vi "Get Service.vi"(7 "Service Type":refnum<class "Service.lvclass">, 8 "error in (no error)":errorcluster, 11 "Values in":refnum<class "Values.lvclass">) -> (0 "error out":errorcluster, 2 "Service":refnum<class "Service.lvclass">, 3 "Values out":refnum<class "Values.lvclass">)   [LabVIEW 2020, in "HTTP Server.lvlib" / "Values.lvclass"]
uses:
  Values.lvclass
  Values.lvclass/Values.ctl
  Service/Service.lvclass
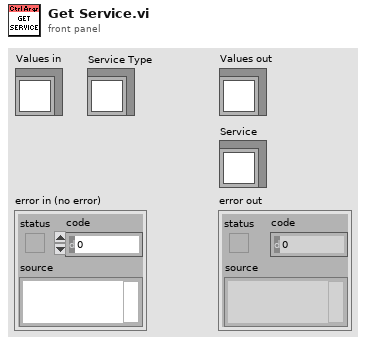
[diagram p1: front panel]
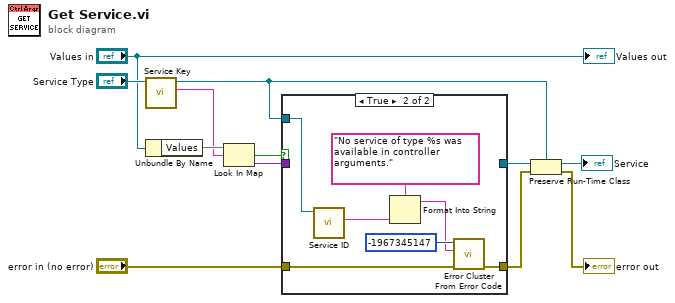
[diagram p0: block diagram]
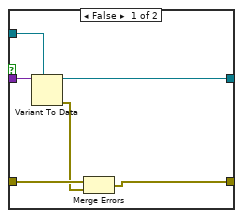
[diagram p2: hidden frame]
diagram:
  n1 = call "Service Key.vi"("Service In"="Service Type") -> ("Service Key"=w9:string, "Service"=w4:refnum<class "Service.lvclass">)  [unwired: 9 in]
  n2 = Unbundle By Name("Values in") -> ("Values"=w10:map{string, variant})
  n3 = Look In Map(map=w10, key=w9) -> (key not found?=w7:bool, value=w6:variant)  [unwired: 1 in]
  n4 = case shown="True" w7 {
    tunnel: w6 -> [w18 _]
    tunnel: "error in (no error)" -> [w15 w22]
    tunnel: [w13 w21] -> w2
    tunnel: w4 -> [w17 w19]
    tunnel: [w16 _] -> w5
    frame False {
      n5 = Variant To Data(type=w17, Variant=w18) -> (data=w16:refnum<class "Service.lvclass">, error out=w14:errorcluster)  [unwired: 1 in]
      n6 = Merge Errors(w15, w14) -> (w13:errorcluster)
    }
    frame True {
      n7 = call-dynamic "Service ID.vi"("Service in"=w19) -> ("Service ID"=w20:string)  [unwired: 8 in, 2 out]
      n8 = Format Into String(format string="No service of type %s was available in controller arguments.", w20) -> (resulting string=w24:string)  [unwired: 2 in, 1 out]
      n9 = call <vilib>:"Error Cluster From Error Code.vi"("error in (no error)"=w22, "error message (\"\")"=w24, "error code (0)"=-1967345147) -> ("error out"=w21:errorcluster)  [unwired: 6 in]
    }
  }
  n10 = Preserve Run-Time Class(object in=w5, error in=w2, 2:w4) -> (object out=→"Service":refnum<class "Service.lvclass">, error out=→"error out":errorcluster)
  "Values out" <- "Values in"
